vi "clear Log.vi"(8 "error in (no error)":errorcluster) -> (0 "error out":errorcluster)   [LabVIEW 2019, in "libConvectionDiffusionWrapper.lvlib"]
doc: "void clearLog();"
uses:
  libConvectionDiffusionWrapper.lvlib
  libConvectionDiffusionWrapper.so
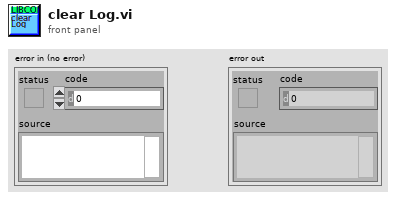
[diagram p1: front panel]
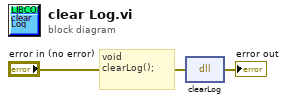
[diagram p0: block diagram]
diagram:
  # "void clearLog();"
  n1 = dll-call lib="home/paul/Schreibtisch/Convection_diffusion/LabView/lib/libConvectionDiffusionWrapper.*" fn="clearLog"(error in="error in (no error)") -> (error out=→"error out":errorcluster)  [unwired: 3 in, 1 out]
